vi "Verify With Regex Scrubber.vi"(11 "LUnit Test Case In":refnum<class "Test Case.lvclass">) -> (0 "error out":errorcluster, 3 "LUnit Test Case Out":refnum<class "Test Case.lvclass">)   [LabVIEW 2020, in "Scrubber Tests.lvclass"]
uses:
  Scrubber Tests.lvclass
  <vilib>/Astemes/LUnit/Test Case.lvclass
  Source/Approval Tests/Options/Options.lvclass
  Source/Approval Tests/Regex Scrubber/Regex Scrubber.lvclass
  Source/Approval Tests/Scrubber/Scrubber.lvclass
  Source/Approval Tests/Namer/Namer.lvclass
  Source/Approval Tests/Naming Data/Naming Data.lvclass
  Source/Approval Tests/Reporter/Reporter.lvclass
  Source/Approval Tests/Text Comparator/Text Comparator.lvclass
  Scrubber Tests.lvclass/Scrubber Tests.ctl
  d22741b7-9abc-4f28-b51a-54e5e2d59af2.vi
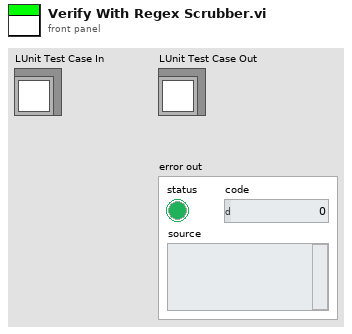
[diagram p1: front panel]
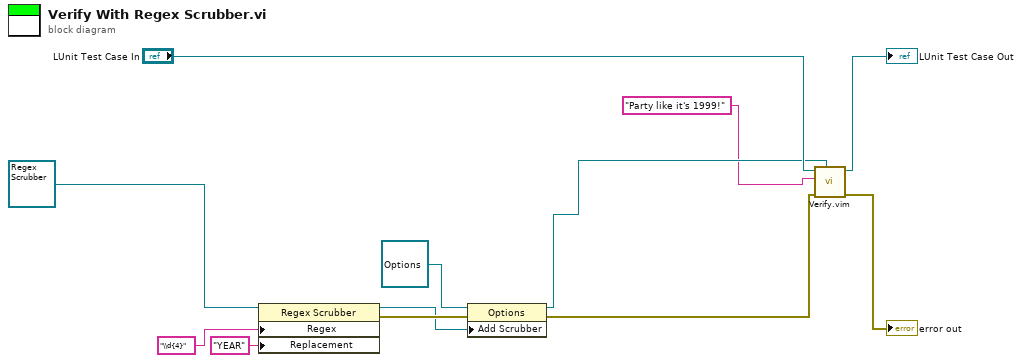
[diagram p0: block diagram]
diagram:
  n1 = property on="Property Node" class="Regex Scrubber"(reference=refnum<class "Regex Scrubber.lvclass"> refnum ("Approval Tests.lvlib:Regex Scrubber.lvclass"), "Regex"="\\d{4}", "Replacement"="YEAR") -> (reference out=w6:refnum<class "Regex Scrubber.lvclass">, error out=w9:errorcluster)  [unwired: 1 in]
  n2 = property class="Options"(reference=refnum<class "Options.lvclass"> refnum ("Approval Tests.lvlib:Options.lvclass"), error in=w9, "Add Scrubber"=w6) -> (reference out=w4:refnum<class "Options.lvclass">, error out=w5:errorcluster)
  n3 = call "Verify.vim"("Options"=w4, "error in"=w5, "Test Data"="Party like it's 1999!", "LUnit Test Case In"="LUnit Test Case In") -> ("error out"=→"error out":errorcluster, "LUnit Test Case Out"=→"LUnit Test Case Out":refnum<class "Test Case.lvclass">)  [unwired: 6 in]
